vi "Tulip handler for Outset table.vi"(5 "State":T2(ring), 6 "Table ID":string="dHSsf5FJpFEqYwqNN", 7 "Part ID":string, 8 "error in":errorcluster, 9 "Body":T1, 10 "Authentication":cluster{"Username":string, "Password":string}={"Username"="apikey.2_WNWgDzkcRL7LwQrSC", "Password"="uUTRYqQF2kxie-OG2NdFiDN_Ok5rwnamrdCqWvd0OVz"}, 11 "URL":string="https://outset-medical-staging.tulip.co/") -> (0 "error out":errorcluster, 1 "Status String":string, 2 "Response body":string)   [LabVIEW 2021]
uses:
  <vilib>/addons/_JKI.lib/REST Client/classes/REST Client/REST Client.lvclass
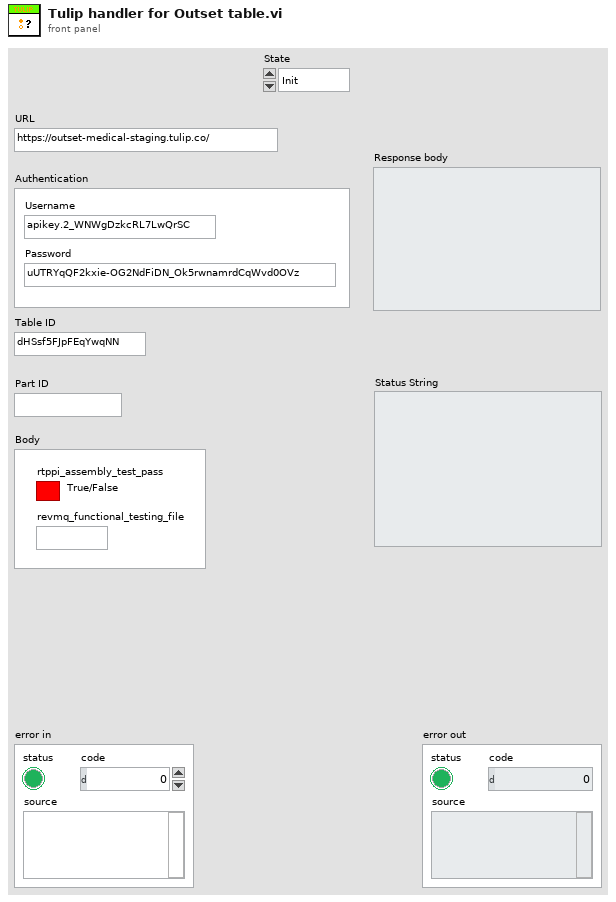
[diagram p1: front panel]
types:
  T1 = cluster{"rtppi_assembly_test_pass":bool, "revmq_functional_testing_file":string}
  T2 = enum16{"Init", "Get headers", "Get", "Post", "Put", "Close"}
  T3 = typedef "REST Client.lvlib/REST Client.lvclass/HTTP Header.ctl" = cluster{"header":string, "value":string}
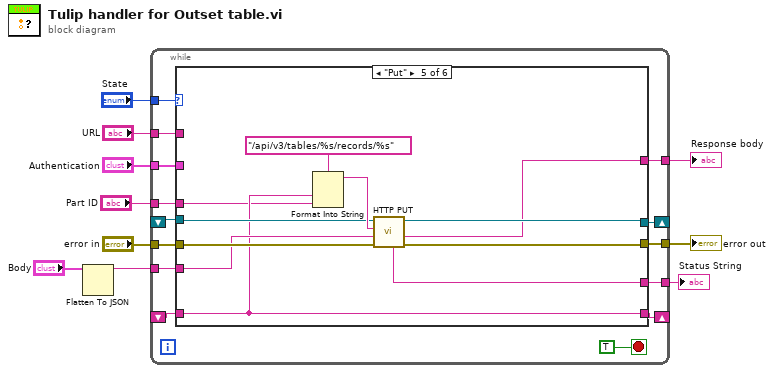
[diagram p0: block diagram]
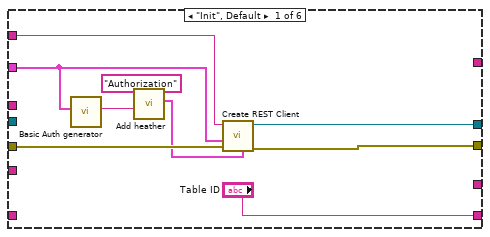
[diagram p2: hidden frame]
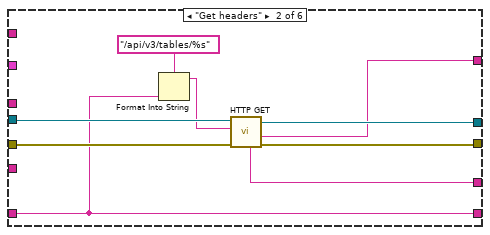
[diagram p3: hidden frame]
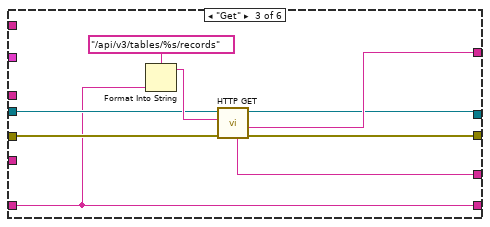
[diagram p4: hidden frame]
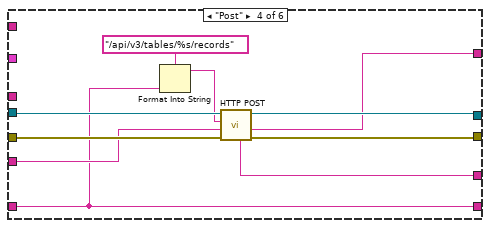
[diagram p5: hidden frame]
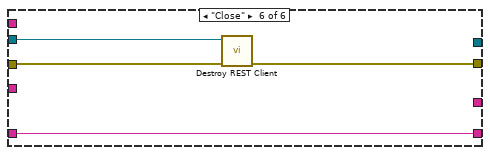
[diagram p6: hidden frame]
diagram:
  n1 = Flatten To JSON(anything="Body") -> (JSON string=w3:string)  [unwired: 2 in, 1 out]
  n2 = while {
    tunnel: "State" -> [w23]
    tunnel: "URL" -> [w22]
    shift-right: [w21] -> _
    shift-left: _ -> [w16]
    tunnel: "Authentication" -> [w20]
    tunnel: "error in" -> [w19]
    tunnel: [w18] -> w6
    tunnel: [w15] -> w5
    tunnel: w3 -> [w14]
    shift-right: [w13] -> _
    shift-left: _ -> [w17]
    tunnel: [w12] -> w2
    tunnel: "Part ID" -> [w11]
    stop <- TRUE stop-if-true
    n3 = case shown="\"Put\"" w23 {
      tunnel: w22 -> [w33 _ _ _ _ _]
      tunnel: [w32 w39 w45 w58 w68 _] -> w21
      tunnel: w20 -> [w29 _ _ _ _ _]
      tunnel: w19 -> [w31 w42 w51 w61 w71 w76]
      tunnel: [w30 w40 w50 w60 w67 w75] -> w18
      tunnel: w17 -> [_ w37 w44 w53 w65 w73]
      tunnel: w16 -> [_ w41 w47 w59 w69 w74]
      tunnel: [_ w38 w46 w54 w66 _] -> w15
      tunnel: w14 -> [_ _ _ w55 w70 _]
      tunnel: ["Table ID" w37 w44 w53 w65 w73] -> w13
      tunnel: [_ w36 w43 w52 w63 _] -> w12
      tunnel: w11 -> [_ _ _ _ w62 _]
      frame "Init", Default {
        n4 = call "Basic Auth generator.vi"("Authentication"=w29) -> ("Basic Auth"=w27:string)  [unwired: 10 in]
        n5 = call "Add heather.vi"("value"=w27, "header"="Authorization") -> ("headers"=w26:T3[])  [unwired: 9 in]
        n6 = call <vilib>:"Create REST Client.vi"("Default Headers ([JSON])"=w26, "error in (no error)"=w31, "Authentication"=w29, "Base URL"=w33) -> ("error out"=w30:errorcluster, "REST Client out"=w32:refnum<class "REST Client.lvclass">)  [unwired: 6 in]
      }
      frame "Get headers" {
        n7 = Format Into String(format string="/api/v3/tables/%s", w37) -> (resulting string=w35:string)  [unwired: 2 in, 1 out]
        n8 = call-dynamic "HTTP GET.vi"("error in (no error)"=w42, "Path"=w35, "REST Client in"=w41) -> ("error out"=w40:errorcluster, "Response body"=w38:string, "REST Client out"=w39:refnum<class "REST Client.lvclass">, "Status String"=w36:string)  [unwired: 3 in, 2 out]
      }
      frame "Get" {
        n9 = Format Into String(format string="/api/v3/tables/%s/records", w44) -> (resulting string=w49:string)  [unwired: 2 in, 1 out]
        n10 = call-dynamic "HTTP GET.vi"("error in (no error)"=w51, "Path"=w49, "REST Client in"=w47) -> ("error out"=w50:errorcluster, "Response body"=w46:string, "REST Client out"=w45:refnum<class "REST Client.lvclass">, "Status String"=w43:string)  [unwired: 3 in, 2 out]
      }
      frame "Post" {
        n11 = Format Into String(format string="/api/v3/tables/%s/records", w53) -> (resulting string=w56:string)  [unwired: 2 in, 1 out]
        n12 = call-dynamic "HTTP POST.vi"("error in (no error)"=w61, "Request body"=w55, "Path"=w56, "REST Client in"=w59) -> ("error out"=w60:errorcluster, "Response body"=w54:string, "REST Client out"=w58:refnum<class "REST Client.lvclass">, "Status String"=w52:string)  [unwired: 2 in, 2 out]
      }
      frame "Put" {
        n13 = Format Into String(format string="/api/v3/tables/%s/records/%s", w65, w62) -> (resulting string=w72:string)  [unwired: 2 in, 1 out]
        n14 = call-dynamic "HTTP PUT.vi"("error in (no error)"=w71, "Request body"=w70, "Path"=w72, "REST Client in"=w69) -> ("error out"=w67:errorcluster, "Response body"=w66:string, "REST Client out"=w68:refnum<class "REST Client.lvclass">, "Status String"=w63:string)  [unwired: 2 in, 2 out]
      }
      frame "Close" {
        n15 = call-dynamic "Destroy REST Client.vi"("error in (no error)"=w76, "REST Client in"=w74) -> ("error out"=w75:errorcluster)  [unwired: 9 in]
      }
    }
  }
  "error out" <- w6
  "Response body" <- w5
  "Status String" <- w2
